vi "ROS_Topic_Read.vi"(3 "ROS in":T1) -> (0 "Reply":string, 1 "ROS out":T1)   [LabVIEW 2013]
doc: "Returns any data received on the topic/service. Only use for subscribers or service clients. Data will need to be parsed."
uses:
  SubVIs/_ROSControl.ctl
  SubVIs/_ROSDirection.ctl
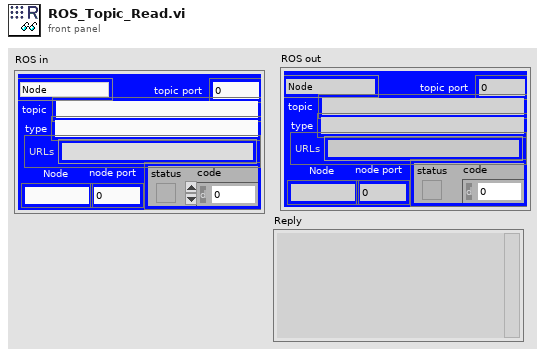
[diagram p1: front panel]
types:
  T1 = typedef "_ROSControl.ctl" = cluster{"topic port":u16, "Node":string, "topic":string, "type":string, "node port":u32, "error ":errorcluster, "Direction":T2, "APIs":string[]}
  T2 = typedef "_ROSDirection.ctl" = enum16{"Node", "Publisher", "Subscriber", "Service Client"}
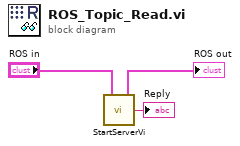
[diagram p0: block diagram]
diagram:
  n1 = call "StartServerVi.vi"("Baxter"="ROS in") -> ("Reply"=→"Reply":string, "Baxter out"=→"ROS out":T1)  [unwired: 1 out]
